vi "Gamma Noise.vi"(7 "initialize?":bool=TRUE, 9 "seed":i32=-1, 10 "order":i32=1, 11 "samples":i32=128) -> (0 "error":i32, 3 "gamma noise":dbl[](array[numeric]))   [LabVIEW 2014, in "NI_AALBase.lvlib"]
doc: "Generates a pseudorandom pattern of values that are the waiting times to the <B>order</B> number event of a unit mean Poisson process."
uses:
  NI_AALBase.lvlib
  lvanlys.dll
panel:
  # "Gamma Noise"
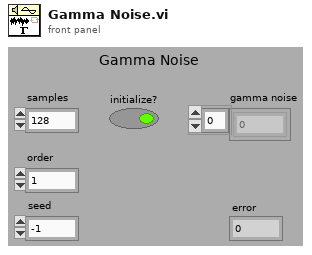
[diagram p1: front panel]
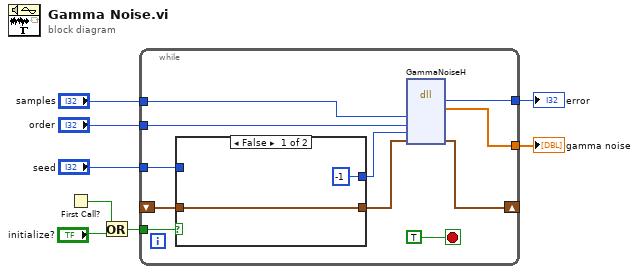
[diagram p0: block diagram]
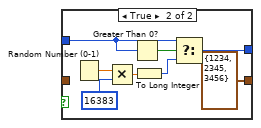
[diagram p2: hidden frame]
diagram:
  n1 = First Call?() -> (First Call?: T/F=w3:bool)
  n2 = Or(x=w3, y="initialize?") -> (x .or. y?=w1:bool)
  n3 = while {
    tunnel: [w16] -> w8
    tunnel: "seed" -> [w15]
    tunnel: "order" -> [w19]
    tunnel: "samples" -> [w18]
    shift-right: [w11] -> _
    shift-left: _ -> [w13]
    tunnel: w1 -> [w10]
    tunnel: [w9] -> w4
    stop <- TRUE stop-if-true
    n4 = case shown="False" w10 {
      tunnel: w13 -> [w21 _]
      tunnel: [w21 cluster{"xSeed":i32, "ySeed":i32, "zSeed":i32} {"xSeed"=1234, "ySeed"=2345, "zSeed"=3456} ("RNGState")] -> w12
      tunnel: [-1 ("seed") w27] -> w14
      tunnel: w15 -> [_ w28]
      frame False {
      }
      frame True {
        n5 = Random Number (0-1)() -> (number: 0 to 1=w25:dbl)
        n6 = Multiply(x=w25, y=16383 ("x")) -> (x*y=w26:dbl)
        n7 = Greater Than 0?(x=w28) -> (x > 0?=w29:bool)
        n8 = To Long Integer(number=w26) -> (32bit integer=w24:i32)
        n9 = Select(t=w28, s=w29, f=w24) -> (s? t:f=w27:i32)
      }
    }
    n10 = dll-call lib="C:/Program Files (x86)/National Instruments/LabVIEW 2014/resource/lvanlys.*" fn="GammaNoiseH"("size"=w18, "order"=w19, "theSeed"=w14, "rngState"=w12) -> ("return type"=w16:i32, "xH"=w9:dbl[], "rngState"=w11:cluster{"xSeed":i32, "ySeed":i32, "zSeed":i32})  [unwired: 6 in, 3 out]
  }
  "error" <- w8
  "gamma noise" <- w4
